vi "DAQmx Start Trigger (Digital Edge).vi"(0 "task/channels in":refnum<k21>, 5 "source":tag, 7 "edge":i32(ring)=10280 items=["Rising"=10280, "Falling"=10171], 11 "error in":errorcluster) -> (4 "task out":refnum<k21>, 15 "error out":errorcluster)   [LabVIEW 2020]
doc: "Configures the task to start acquiring or generating samples on a rising or falling edge of a digital signal."
uses:
  nilvaiu.dll
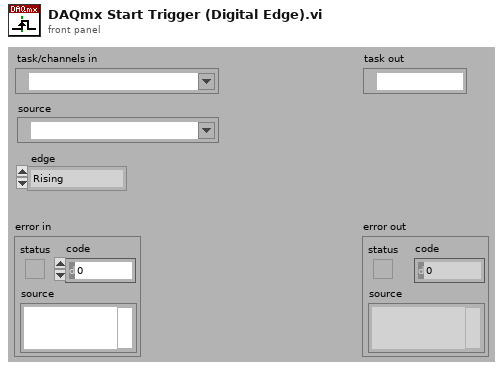
[diagram p1: front panel]
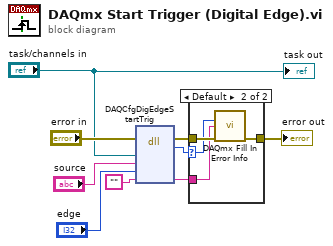
[diagram p0: block diagram]
diagram:
  n1 = dll-call lib="nilvaiu.*" fn="DAQCfgDigEdgeStartTrig"(error in="error in", "taskID"="task/channels in", "source"="source", "edge"="edge", "extendedErrorIndo"="") -> (error out=w3:errorcluster, "return type"=w4:i32, "extendedErrorIndo"=w2:string)  [unwired: 5 in, 1 out]
  n2 = case shown="Default" w4 {
    selector: w4 -> [_ w12]
    tunnel: w3 -> [w10 w14]
    tunnel: [w10 w13] -> w8
    tunnel: w2 -> [_ w11]
    frame 0 {
    }
    frame Default {
      n3 = call "DAQmx Fill In Error Info.vi"("status code"=w12, "extended error info"=w11, "error in"=w14) -> ("error out"=w13:errorcluster)  [unwired: 1 in, 11 out]
    }
  }
  "error out" <- w8
  "task out" <- "task/channels in"
